vi "FlatToRichsift_proxy_v1_ChannelEnumType.vi"(5 "OutputClusterType":T1, 11 "InputCluster":T2) -> (3 "OutputCluster":T1)   [LabVIEW 2024, in "SiftProxy_client.lvlib"]
uses:
  sift_proxy_v1_ChannelEnumType_Flat.ctl
  sift_proxy_v1_ChannelEnumType.ctl
  SiftProxy_client.lvlib
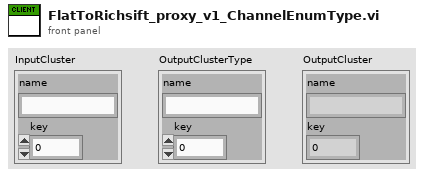
[diagram p1: front panel]
types:
  T1 = typedef "SiftProxy_client.lvlib/sift_proxy_v1_ChannelEnumType.ctl" = cluster{"name":string, "key":u32}
  T2 = typedef "SiftProxy_client.lvlib/sift_proxy_v1_ChannelEnumType_Flat.ctl" = cluster{"name":string, "key":u32}
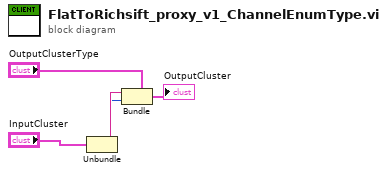
[diagram p0: block diagram]
diagram:
  n1 = Unbundle "Unbundle"("InputCluster") -> ("name"=w2:string, "key"=w1:u32)
  n2 = Bundle "Bundle"(cluster="OutputClusterType", "name"=w2, "key"=w1) -> (→"OutputCluster":T1)
